vi "Apply Mask.vi"(0 "image in":refnum<class "MSC Image.lvclass">, 1 "mask image in":refnum<class "MSC Image.lvclass">, 5 "error in (no error)":errorcluster) -> (14 "image out":refnum<class "MSC Image.lvclass">, 15 "mask image out":refnum<class "MSC Image.lvclass">, 19 "error out":errorcluster)   [LabVIEW 2016, in "MSC Image.lvclass"]
doc: "Applies a mask to the image which only leaves \"marked\" pixels and sets the other ones to 0.\nAll pixels unequal to 0 in the mask image are \"marked\"."
uses:
  MSC Image.lvclass
  Dependencies/x86/MSC I Process32.dll
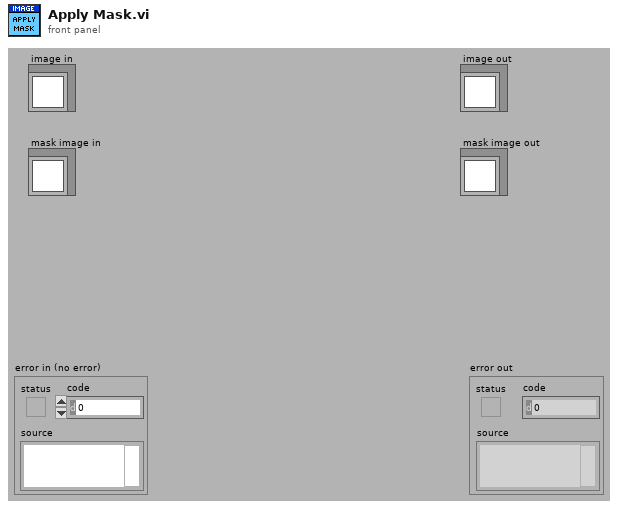
[diagram p1: front panel]
types:
  T1 = typedef "Image.ctl" = cluster{"Pointer":u64, "Size":T2, "Image Type":T3, "Time Stamp":timestamp, "Variant":variant}
  T2 = typedef "Size.ctl" = cluster{"Cols":i32, "Rows":i32}
  T3 = typedef "Image Type.ctl" = i32
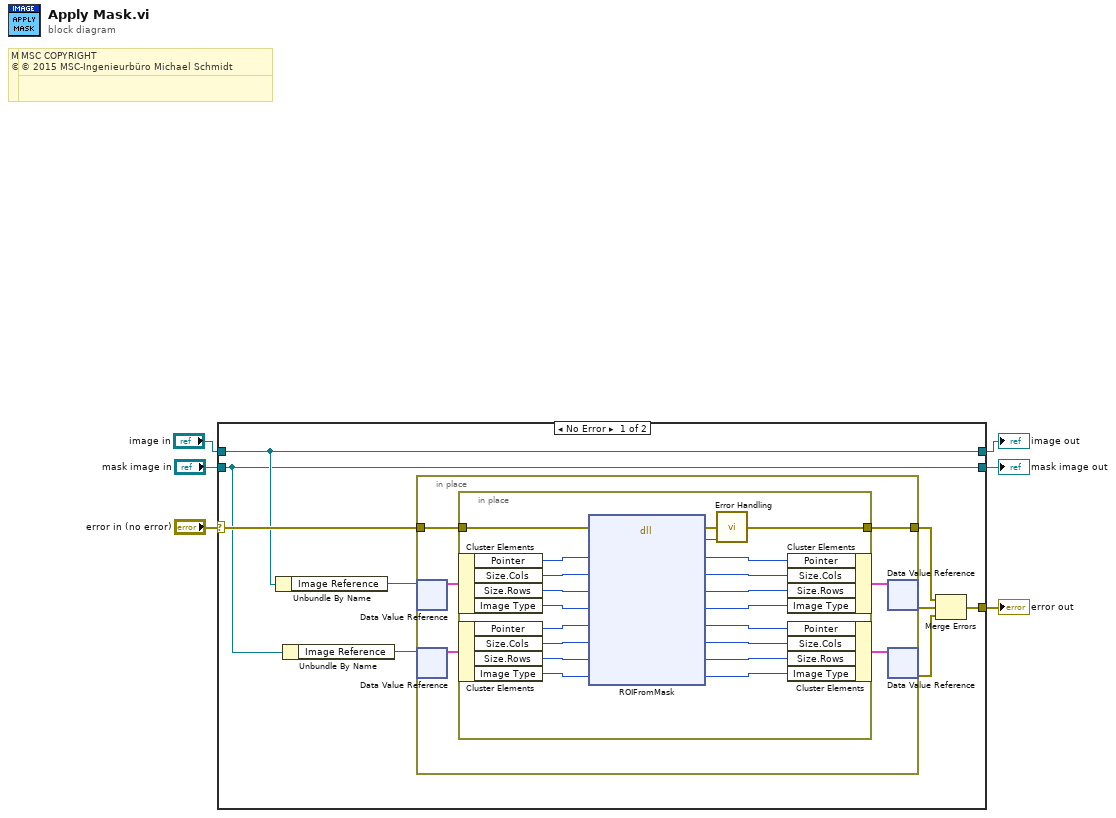
[diagram p0: block diagram]
diagram:
  # "MSC COPYRIGHT\n© 2016 MSC-Ingenieurbüro Michael Schmidt"
  # "MSC COPYRIGHT\n© 2016 MSC-Ingenieurbüro Michael Schmidt"
  # "MSC COPYRIGHT\n© 2015 MSC-Ingenieurbüro Michael Schmidt"
  # "MSC COPYRIGHT\n© 2015 MSC-Ingenieurbüro Michael Schmidt"
  n1 = case shown="No Error" "error in (no error)" {
    selector: "error in (no error)" -> [w11 w44]
    tunnel: [w15 w44] -> w2
    tunnel: [w7 w43] -> w5
    tunnel: "image in" -> [w10 w42]
    tunnel: "mask image in" -> [w7 w43]
    tunnel: [w10 w42] -> w6
    frame No Error {
      n2 = Unbundle By Name(w10) -> ("Image Reference"=w9:refnum<data-value>)
      n3 = Unbundle By Name(w7) -> ("Image Reference"=w8:refnum<data-value>)
      n4 = in-place {
        in-place-border: w11 -> [w19]
        in-place-border: [w18] -> w14
        n5 = in-place-dvr #1(w9) -> (w20:T1)  [unwired: 1 out]
        n6 = in-place-dvr #2(w8) -> (w17:T1)  [unwired: 1 out]
        n7 = in-place {
          in-place-border: w19 -> [w22]
          in-place-border: [w41] -> w18
          n8 = in-place-cluster #3(w20) -> ("Pointer"=w40:u64, "Size.Cols"=w39:i32, "Size.Rows"=w38:i32, "Image Type"=w37:T3)
          n9 = in-place-cluster #4(w17) -> ("Pointer"=w36:u64, "Size.Cols"=w35:i32, "Size.Rows"=w34:i32, "Image Type"=w33:T3)
          n10 = dll-call lib="C:/Users/MSC/LabVIEW Projekte/LV 2014/MSC I-Process/user.lib/MSC-I Process/Dependencies/x86/MSC I Process*.dll" fn="ROIFromMask"(error in=w22, "pointer"=w40, "cols"=w39, "rows"=w38, "type"=w37, "pointerMask"=w36, "colsMask"=w35, "rowsMask"=w34, "typeMask"=w33) -> (error out=w23:errorcluster, "error"=w24:i32, "pointer"=w28:u64, "cols"=w27:i32, "rows"=w26:i32, "type"=w25:i32, "pointerMask"=w32:u64, "colsMask"=w31:i32, "rowsMask"=w30:i32, "typeMask"=w29:i32)  [unwired: 2 in, 1 out]
          n11 = call "Error Handling.vi"("error in (no error)"=w23, "return type"=w24) -> ("error out"=w41:errorcluster)  [unwired: 12 in, 1 out]
          n12 = in-place-cluster #3("Pointer"=w28, "Size.Cols"=w27, "Size.Rows"=w26, "Image Type"=w25) -> (w21:T1)
          n13 = in-place-cluster #4("Pointer"=w32, "Size.Cols"=w31, "Size.Rows"=w30, "Image Type"=w29) -> (w16:T1)
        }
        n14 = in-place-dvr #1(w21) -> (w13:errorcluster)  [unwired: 1 out]
        n15 = in-place-dvr #2(w16) -> (w12:errorcluster)  [unwired: 1 out]
      }
      n16 = Merge Errors(w14, w13, w12) -> (w15:errorcluster)
    }
    frame Error {
    }
  }
  "error out" <- w2
  "image out" <- w6
  "mask image out" <- w5
